vi "Fill_Combo_API_Box (SubVI).vi"(6 "Section Name":string="Publish Topic", 7 "Key Name":string="Topics", 9 "Combo Box":string(combo)="test/CPU/CPUcommand", 10 "configuration file path":path=path "D:/James Pratice LV/MQTT.ini", 11 "ComboBox in":refnum<vi>) -> ()   [LabVIEW 2018]
uses:
  <vilib>/Utility/config.llb/Read Key (String).vi
  <vilib>/Utility/config.llb/NI_LVConfig.lvlib
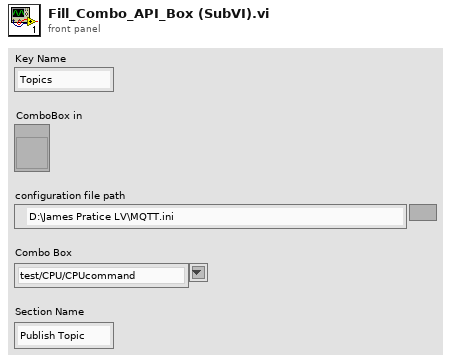
[diagram p1: front panel]
types:
  T1 = typedef "NI_LVConfig.lvlib/Config Data RefNum.ctl" = refnum<k1>
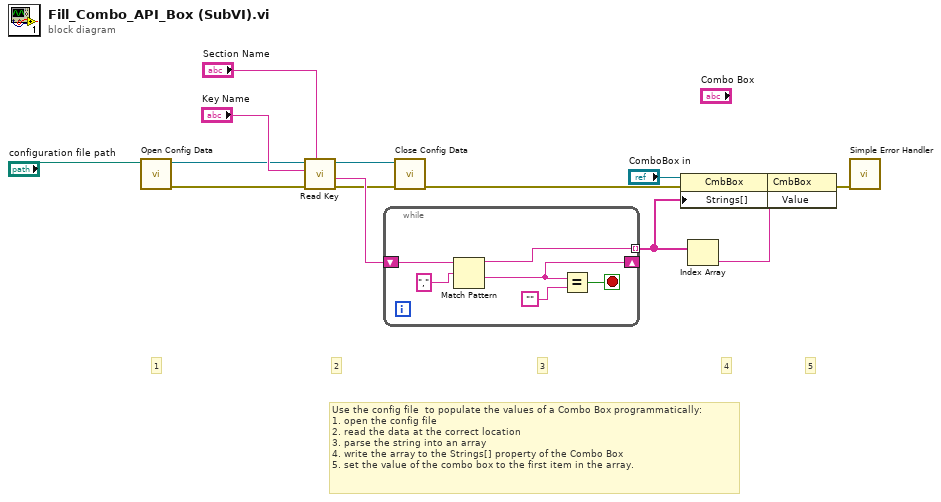
[diagram p0: block diagram]
diagram:
  # "5"
  # "4"
  # "3"
  # "2"
  # "1"
  # "Use the config file  to populate the values of a Combo Box programmatically:\n1. open the config file\n2. read the data at the correct location\n3. parse the string into an array\n4. write the array to the Strings[] property of the Combo Box\n5. set the value of the combo box to the first item in the array."
  n1 = call <vilib>:"Open Config Data.vi"("configuration file path"="configuration file path") -> ("error out"=w3:errorcluster, "refnum"=w2:T1)  [unwired: 8 in, 1 out]
  n2 = call-poly <vilib>:"Read Key.vi"("section"="Section Name", "error in (no error)"=w3, "key"="Key Name", "refnum"=w2) -> ("error out"=w7:errorcluster, "value"=w8:string, "refnum out"=w6:T1)  [unwired: 4 in, 1 out]
  n3 = while {
    tunnel: [w16] -> w9 mode=indexing
    shift-right: [w15] -> _
    shift-left: w8 -> [w20]
    stop <- w17 stop-if-true
    n4 = Match Pattern(string=w20, regular expression=",") -> (before substring=w16:string, after substring=w15:string)  [unwired: 1 in, 2 out]
    n5 = Equal?(x=w15, y="") -> (x = y?=w17:bool)
  }
  n6 = call <vilib>:"Close Config Data.vi"("error in (no error)"=w7, "refnum"=w6) -> ("error out"=w13:errorcluster)  [unwired: 8 in, 1 out]
  n7 = property on="Property Node" class="CmbBox"(reference="ComboBox in", error in=w13, "Strings[]"=w9) -> (error out=w12:errorcluster)  [unwired: 1 out]
  n8 = Index Array "Index Array"(array=w9) -> (element=w10:string)  [unwired: 1 in]
  n9 = property on="Property Node" class="CmbBox"(reference="ComboBox in", error in=w12, "Value"=w10) -> (error out=w11:errorcluster)  [unwired: 1 out]
  n10 = call <vilib>:"Simple Error Handler.vi"("error in (no error)"=w11) -> ()  [unwired: 4 in, 5 out]
